vi "udp_saatja.vi"() -> ()   [LabVIEW 2020]
panel:
  in  "Send":bool
  in  "tekst":string
  in  "Stop":bool
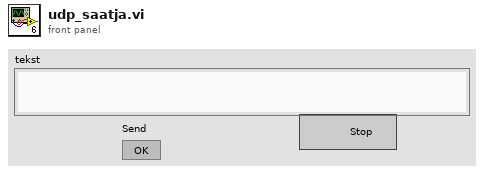
[diagram p1: front panel]
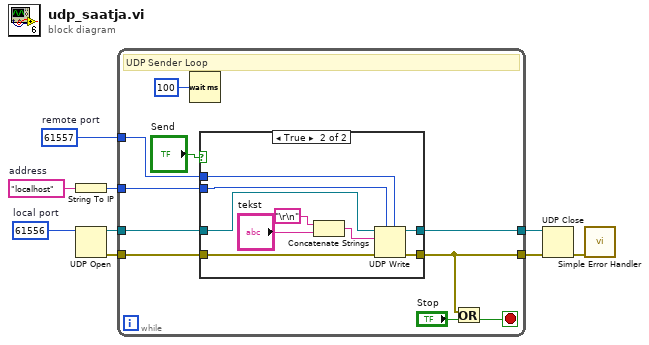
[diagram p0: block diagram]
diagram:
  w1 = u16 61557  # remote port
  w2 = u16 61556  # local port
  w7 = "localhost"  # address
  n1 = String To IP(1:w7) -> (0:w5:u32)
  n2 = UDP Open(11:w2) -> (port=w4:refnum<k16>, 0:w3:errorcluster)  [unwired: 4 in, 1 out]
  n3 = while {
    tunnel: [w14] -> w8
    tunnel: w4 -> [w19]
    tunnel: w3 -> [w18]
    tunnel: [w15] -> w9
    tunnel: w5 -> [w13]
    tunnel: w1 -> [w11]
    stop <- w17 stop-if-true
    # "UDP Sender Loop"
    n4 = Wait (ms)(milliseconds to wait=u32 100) -> ()  [unwired: 1 out]
    n5 = case shown="True" "Send" {
      tunnel: w19 -> [w21 w30]
      tunnel: w18 -> [w20 w29]
      tunnel: [w21 w28] -> w15
      tunnel: [w20 w27] -> w14
      tunnel: w13 -> [_ w26]
      tunnel: w11 -> [_ w25]
      frame False {
      }
      frame True {
        n6 = Concatenate Strings("\r\n", "tekst") -> (w22:string)
        n7 = UDP Write(address=w26, port or service name=w25, connection ID=w30, data in=w22, 8:w29) -> (error out=w27:errorcluster, 3:w28:refnum<k16>)  [unwired: 1 in]
      }
    }
    n8 = Or(x=w14, y="Stop") -> (x .or. y?=w17:bool)
  }
  n9 = UDP Close(connection ID=w9, 8:w8) -> (error out=w6:errorcluster)  [unwired: 1 out]
  n10 = call <vilib>:"Simple Error Handler.vi"("error in (no error)"=w6) -> ()  [unwired: 4 in, 5 out]
